vi "Read Wait Until Done_.vi"(8 "error in (no error)":errorcluster, 11 "Run VI in":refnum<class "Run VI.lvclass">) -> (0 "error out":errorcluster, 2 "Wait Until Done?":bool, 3 "Run VI out":refnum<class "Run VI.lvclass">)   [LabVIEW 2014, in "Run VI.lvclass"]
uses:
  Run VI.lvclass
  Run VI.lvclass/Run VI.ctl
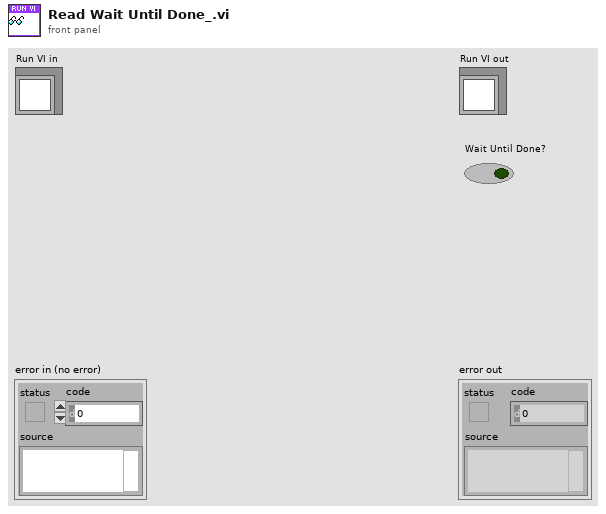
[diagram p1: front panel]
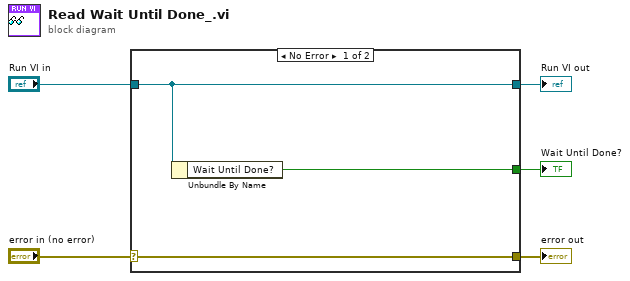
[diagram p0: block diagram]
diagram:
  n1 = case shown="No Error" "error in (no error)" {
    selector: "error in (no error)" -> [w8 w9]
    tunnel: [w8 w9] -> w4
    tunnel: [w7 w10] -> w2
    tunnel: "Run VI in" -> [w7 w10]
    tunnel: [w6 _] -> w1
    frame No Error {
      n2 = Unbundle By Name(w7) -> ("Wait Until Done?"=w6:bool)
    }
    frame Error {
    }
  }
  "error out" <- w4
  "Run VI out" <- w2
  "Wait Until Done?" <- w1
